vi "Main.vi"(8 "error in (no error)":errorcluster, 11 "Control VI":T1) -> (0 "error out":errorcluster)   [LabVIEW 2020, in "FormulaG.lvlib" / "FormulaG App.lvclass"]
uses:
  FormulaG App.lvclass
  FormulaLV-Common/Control VI.ctl
  FormulaLV-Common/FormulaG-Common.lvlib
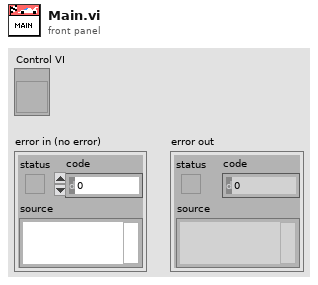
[diagram p1: front panel]
types:
  T1 = typedef "FormulaG-Common.lvlib/Control VI.ctl" = refnum<vi>
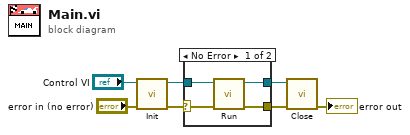
[diagram p0: block diagram]
diagram:
  n1 = call "Init.vi"("error in (no error)"="error in (no error)", "Control VI"="Control VI") -> ("error out"=w7:errorcluster, "FormulaLV App out"=w6:refnum<class "FormulaG App.lvclass">)  [unwired: 8 in]
  n2 = case shown="No Error" w7 {
    selector: w7 -> [w10 w13]
    tunnel: w6 -> [w11 w12]
    tunnel: [w9 w13] -> w5
    tunnel: [w8 w12] -> w4
    frame No Error {
      n3 = call "Run.vi"("error in (no error)"=w10, "FormulaLV App in"=w11) -> ("error out"=w9:errorcluster, "FormulaLV App out"=w8:refnum<class "FormulaG App.lvclass">)  [unwired: 8 in]
    }
    frame Error {
    }
  }
  n4 = call "Close.vi"("error in (no error)"=w5, "FormulaLV App in"=w4) -> ("error out"=→"error out":errorcluster)  [unwired: 9 in]
